vi "Swap Controllers.vi"(8 "error in (no error)":cluster{"状态":bool, "代码":i32, "源":string} caption="错误输入（无错误）", 10 "冷却器控制器":refnum<class "Cooler Controller.lvclass">, 11 "气冷系统应用程序输入":refnum<class "Air Cooler Application.lvclass">) -> (0 "error out":cluster{"状态":bool, "代码":i32, "源":string} caption="错误输出", 3 "气冷系统应用程序输出":refnum<class "Air Cooler Application.lvclass">)   [LabVIEW 2015, in "Air Cooler Application.lvlib" / "Air Cooler Application.lvclass"]
doc: "本VI负责更改当前正在运行的控制器操作者。输入的控制器将被启动，当前控制器将被停止。切换过程中冷却器将保持运行状态，不会被中断。"
uses:
  Air Cooler Application.lvclass
  Cooler Controller/Cooler Controller/Cooler Controller.lvclass
  <vilib>/ActorFramework/Message Enqueuer/Message Enqueuer.lvclass
  <vilib>/ActorFramework/Message Enqueuer/Message Priority.ctl
  Air Cooler Application.lvclass/Air Cooler Application.ctl
  Cooler Controller/Write Cooler Enqueuer Msg/Write Cooler Enqueuer Msg.lvclass/Write Cooler Enqueuer Msg.ctl
  <vilib>/ActorFramework/Message Enqueuer/Message Enqueuer.lvclass/Message Enqueuer.ctl
  Cooler/Write Controller Enqueuer Msg/Write Controller Enqueuer Msg.lvclass/Write Controller Enqueuer Msg.ctl
  <vilib>/ActorFramework/Message Enqueuer/Enqueue.vi
  <vilib>/ActorFramework/Message Priority Queue/Priority Enqueue.vi
  Cooler Controller/Write Cooler Enqueuer Msg/Write Cooler Enqueuer Msg.lvclass
  Cooler/Write Controller Enqueuer Msg/Write Controller Enqueuer Msg.lvclass
  <vilib>/ActorFramework/Stop Msg/Stop Msg.lvclass
  <vilib>/ActorFramework/Actor/Actor.lvclass
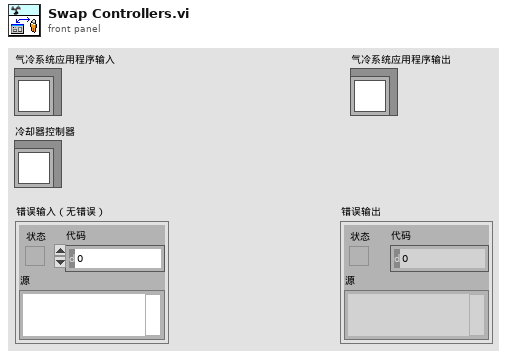
[diagram p1: front panel]
types:
  T1 = typedef "Actor Framework.lvlib/Message Enqueuer.lvclass/Message Priority.ctl" = enum16{"Low", "Normal", "High"}
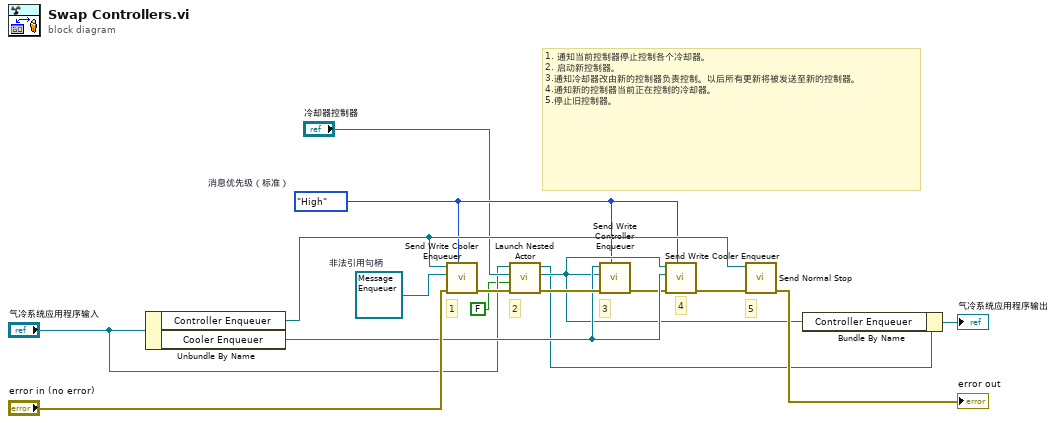
[diagram p0: block diagram]
diagram:
  w5 = Message_Priority."High"  # 消息优先级（标准）
  w12 = refnum<class "Message Enqueuer.lvclass"> refnum  # 非法引用句柄
  # "4"
  # "1. 通知当前控制器停止控制各个冷却器。\n2. 启动新控制器。\n3.通知冷却器改由新的控制器负责控制。以后所有更新将被发送至新的控制器。\n4.通知新的控制器当前正在控制的冷却器。\n5.停止旧控制器。"
  # "5"
  # "3"
  # "2"
  # "1"
  n1 = Unbundle By Name("气冷系统应用程序输入") -> ("Controller Enqueuer"=w10:refnum<class "Message Enqueuer.lvclass">, "Cooler Enqueuer"=w9:refnum<class "Message Enqueuer.lvclass">)
  n2 = call "Send Write Cooler Enqueuer.vi"("消息优先级（标准）"=w5, "error in (no error)"="error in (no error)", "冷却器待入队列"=w12, "消息待入队列"=w10) -> ("error out"=w13:cluster{"状态":bool, "代码":i32, "源":string})  [unwired: 7 in]
  n3 = call <vilib>:"Launch Nested Actor.vi"("error in (no error)"=w13, "Auto-stop? (T)"=FALSE, "Nested Actor"="冷却器控制器", "Caller Actor in"="气冷系统应用程序输入") -> ("error out"=w11:errorcluster, "Nested Actor's Enqueuer"=w8:refnum<class "Message Enqueuer.lvclass">, "Caller Actor out"=w2:refnum<class "Air Cooler Application.lvclass">)  [unwired: 5 in]
  n4 = call "Send Write Controller Enqueuer.vi"("消息优先级（标准）"=w5, "error in (no error)"=w11, "控制器待入队列"=w8, "消息待入队列"=w9) -> ("error out"=w7:cluster{"状态":bool, "代码":i32, "源":string})  [unwired: 7 in]
  n5 = call "Send Write Cooler Enqueuer.vi"("消息优先级（标准）"=w5, "error in (no error)"=w7, "冷却器待入队列"=w9, "消息待入队列"=w8) -> ("error out"=w6:cluster{"状态":bool, "代码":i32, "源":string})  [unwired: 7 in]
  n6 = call <vilib>:"Send Normal Stop.vi"("error in (no error)"=w6, "Message Enqueuer"=w10) -> ("error out"=→"error out":errorcluster)  [unwired: 9 in]
  n7 = Bundle By Name(cluster=w2, "Controller Enqueuer"=w8) -> (→"气冷系统应用程序输出":refnum<class "Air Cooler Application.lvclass">)
